vi "SPI API Main.vi"() -> ()   [LabVIEW 2014]
doc: "This example is based on the MAX5216. It allows you to control the voltage output on the SPI chip. This VI interfaces with the SPI Engine on the FPGA."
uses:
  Source/Shared/MCP23S17/Chip Address.ctl
  Source/Shared/MCP23S17/Pin.ctl
  Source/Shared/MCP23S17/Pin Mode.ctl
  Source/Shared/MCP23S17/IOCON BANK 0 Reg Addresses.ctl
  <vilib>/FPGAPlugInAG/cRIO-9081/niLvFpga_Open_cRIO-9081.vi
  <vilib>/rvi/interface/common/dynamic/niFpgaDynamicAddResources.vi
  <vilib>/FPGAPlugInAG/Dynamic/niLvFpga_Reset_Dynamic.vi
  <vilib>/FPGAPlugInAG/Dynamic/niLvFpga_Run_Dynamic.vi
  <vilib>/Utility/error.llb/Error Cluster From Error Code.vi
  <vilib>/rvi/errors/niLvFpgaAdjustHostInterfaceError.vi
  Source/Shared/MCP23S17/Update Mode All Pins.vi
  Source/Shared/MCP23S17/Write Digital All Pins.vi
  Source/Shared/MCP23S17/Write Digital Pin.vi
  Source/Shared/MCP23S17/Update Mode Pin.vi
  Source/Shared/MCP23S17/Update Output Latch All Pins.vi
  Source/Shared/MCP23S17/Update Input Polarity All Pins.vi
  <vilib>/FPGAPlugInAG/Dynamic/niLvFpga_Close_Dynamic.vi
  <vilib>/rvi/interface/nirviOpenFPGA/nirviOpenFPGA.xnode
  FPGA Bitfiles/SPIAPITest_FPGATarget_SPIAPIFPGA_fdd6JLrBLcE.lvbitx
  <vilib>/rvi/interface/nirviMethod/nirviMethod.xnode
  <vilib>/rvi/interface/nirviReadWriteControl/nirviReadWriteControl.xnode
  <vilib>/rvi/interface/nirviCloseFPGA/nirviCloseFPGA.xnode
  <vilib>/rvi/interface/Simulation/niFpgaSimulationCallBeginRW.vi
  NiFpgaLv.dll
  Source/Shared/SLSC configuration Shared.lvlib
  <vilib>/FPGAPlugInAG/Dynamic/niLvFpga_WriteFifo_Dynamic.vi
  <vilib>/rvi/errors/niLvFpgaMergeErrorWithErrorCode.vi
panel:
  in  "Input Polarity":u16 format="%.0b"
  out "Input Polarity Cache":u16 format="%016b"
  out "Output Latch Cache":u16 format="%016b"
  in  "Output Latch":u16 format="%.0b"
  in  "IOCON.BANK = 0 Reg Addresses":T1
  in  "Pin Mode":T2
  out "NC":u64 format="%.0b"
  in  "Pin Value":u8 format="%.0b"
  in  "Pin":T3=1 min=1 max=16
  out "Mode Cache":u16 format="%016b"
  out "Output Cache":u16 format="%016b"
  in  "Value":u16 format="%016b"
  out "SPI Command":u32 format="%.0b"
  out "Transfer Length (bits)":u8
  in  "Mode":u16 format="%016b"
  in  "Chip Address (A2 A1 A0)":T4 max=7
  in  "Message  Type":T5(ring)
  out "Chip Select out":u8
  out "Data to DAC":u64 format="%032b"
  in  "Write":bool
  in  "Chip Select":u8
  out "Binary to DAC":u64
  in  "data rate (S/s)":u32=4000000
  in  "SPI PHY Settings":T6={"Divide Value"=255, "Transfer Length (bits)"=32, "CS Asserted Polarity"=FALSE, "Clock Polarity (CPOL)"=FALSE, "Clock Phase (CPHA)"=FALSE, "Lengthen MISO Setup"=FALSE, "Direction Change Bit"=0, "MOSI Starts as Output"=FALSE, "Tristatable MOSI"=FALSE}
  in  "stop":bool
  # "Overview: This example is based on the MAX5216.  It allows you to control the\nvoltage output on the SPI chip. \nRequirements: LabVIEW Full Development System, LabVIEW Real Time, \nLabVIEW FPGA, MAX5216, NI System on Module, NI 9651.\nInstructions:\n1. The SPI PHY Settings are already setup for the MAX5216.  Do not adjust them.\n2. Plug the MAX5216 into PMOD1 on the NI 9651.\n3. Setup Vref according to the user manual.\n4. Run the VI.\n5. Adjust the Voltage Output and observe the voltage change on the MAX5216."
  # "SPI Settings"
  # "MSB"
  # "LSB"
  # "Sampling Info"
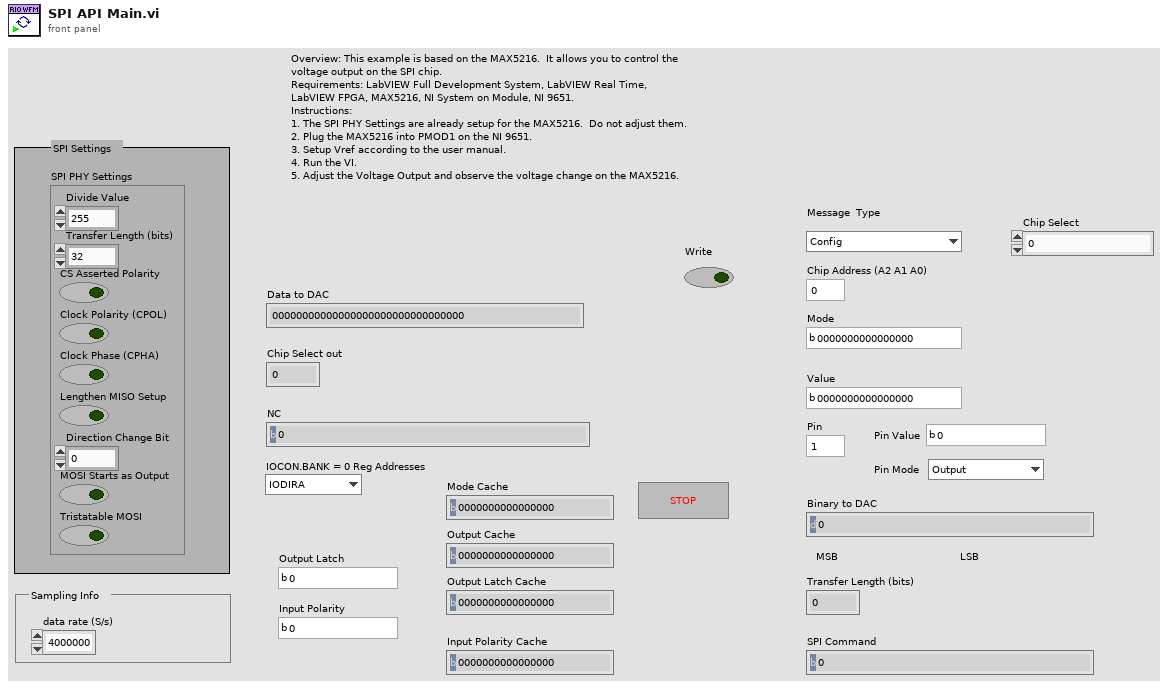
[diagram p1: front panel]
types:
  T1 = typedef "SLSC configuration Shared.lvlib/IOCON BANK 0 Reg Addresses.ctl" = enum8{"IODIRA", "IODIRB", "IPOLA", "IPOLB", "GPINTENA", "GPINTENB", "DEFVALA", "DEFVALB", "INTCONA", "INTCONB", "IOCONA", "IOCONB", "GPPUA", "GPPUB", "INTFA", "INTFB", "INTCAPA", "INTCAPB", "GPIOA", "GPIOB", "OLATA", "OLATB"}
  T2 = typedef "SLSC configuration Shared.lvlib/Pin Mode.ctl" = enum8{"Output", "Input"}
  T3 = typedef "SLSC configuration Shared.lvlib/Pin.ctl" = u8
  T4 = typedef "SLSC configuration Shared.lvlib/Chip Address.ctl" = u8
  T5 = enum16{"Config", "Update Mode All Pins", "Update Mode Pin", "Write Digital All Pins", "Write Digital Pin", "Read Digital Pins", "Read Byte", "Update Output Latches All Pins", "Update Input Polarity All Pins", "Arindam 1", "Arindam 2", "Ardinam 3"}
  T6 = cluster{"Divide Value":u8, "Transfer Length (bits)":u8, "CS Asserted Polarity":bool, "Clock Polarity (CPOL)":bool, "Clock Phase (CPHA)":bool, "Lengthen MISO Setup":bool, "Direction Change Bit":u8, "MOSI Starts as Output":bool, "Tristatable MOSI":bool}
  T7 = typedef "SLSC configuration Shared.lvlib/SPI Command.ctl" = cluster{"SPI Command":u32, "Transfer Length":u8}
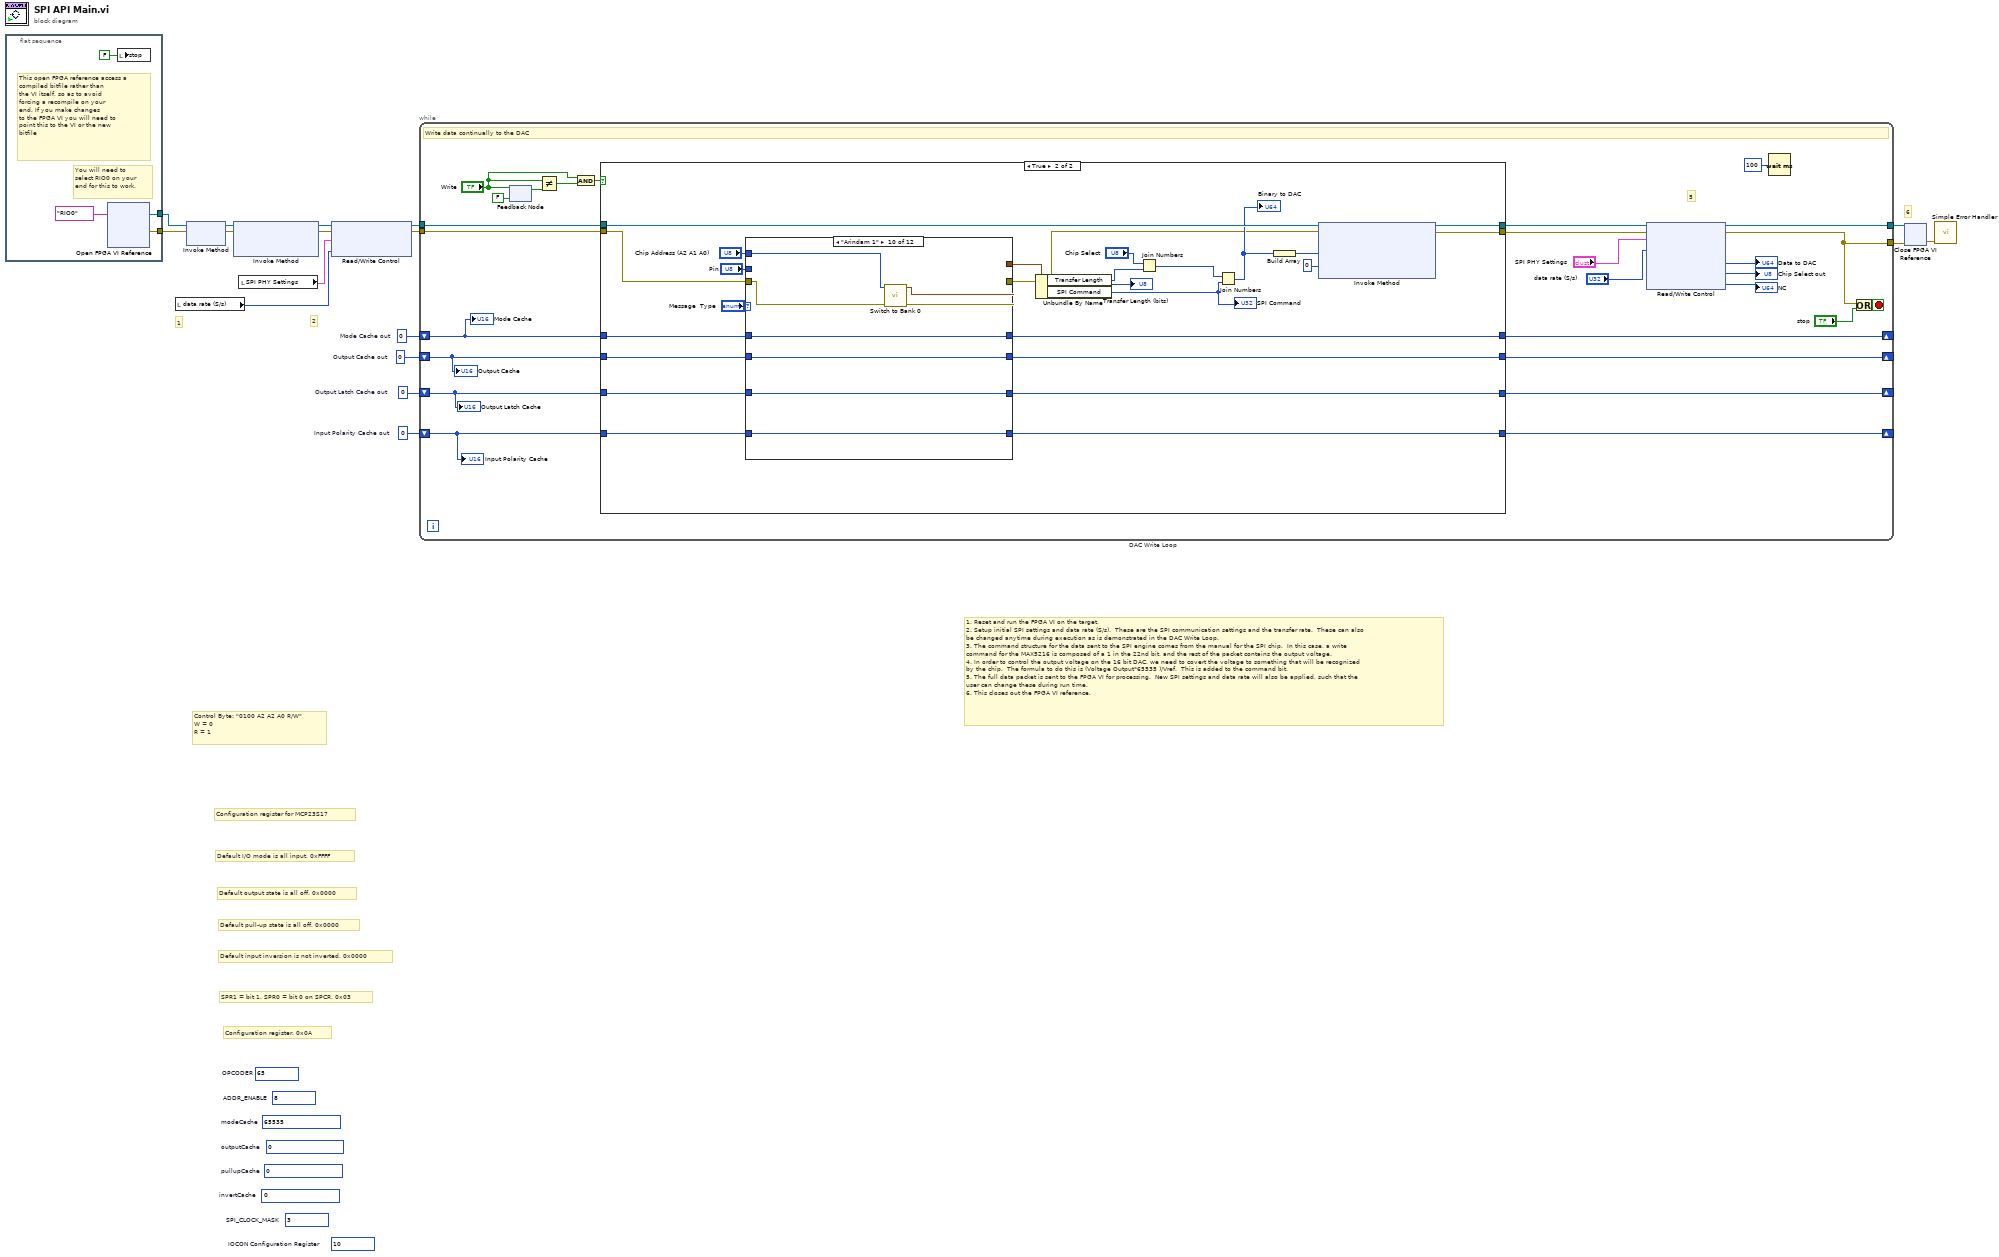
[diagram p0: block diagram]
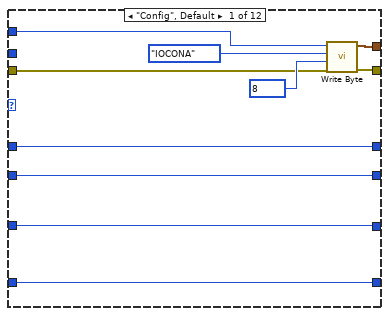
[diagram p3: hidden frame]
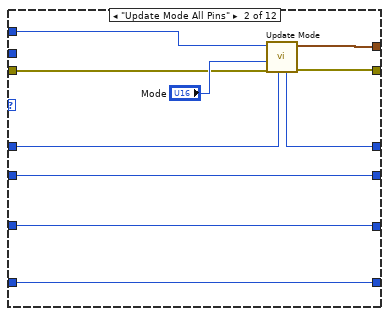
[diagram p4: hidden frame]
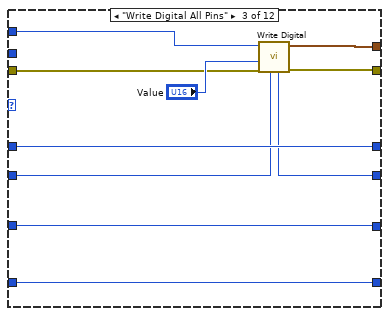
[diagram p5: hidden frame]
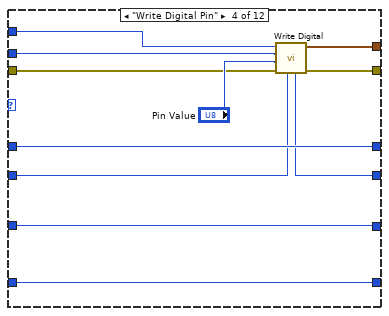
[diagram p6: hidden frame]
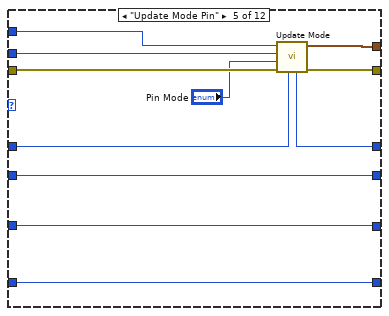
[diagram p7: hidden frame]
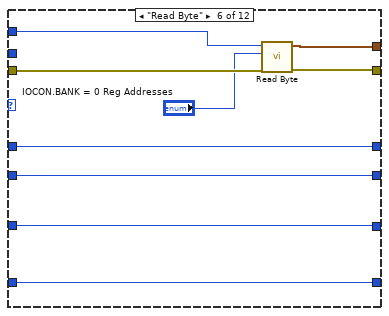
[diagram p8: hidden frame]
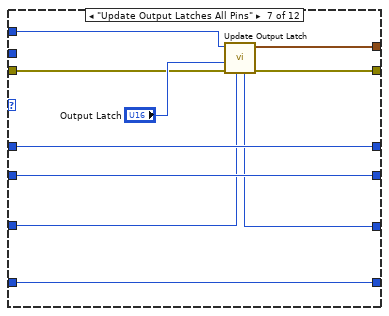
[diagram p9: hidden frame]
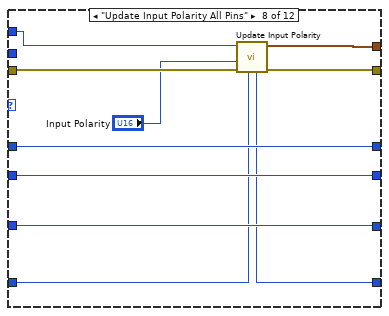
[diagram p10: hidden frame]
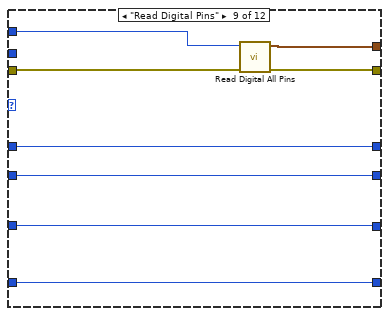
[diagram p11: hidden frame]
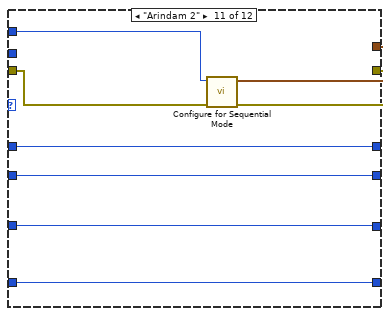
[diagram p12: hidden frame]
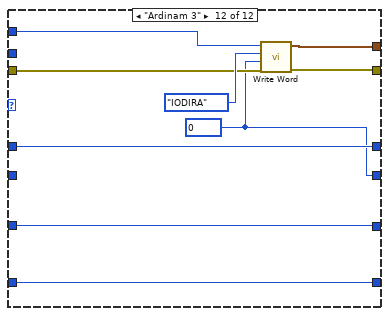
[diagram p13: hidden frame]
diagram:
  w1 = u16 0  # Input Polarity Cache out
  w2 = u16 0  # Output Latch Cache out
  w3 = u16 0  # Output Cache out
  w4 = u16 0  # Mode Cache out
  (unwired) u8 10  # IOCON Configuration Register
  (unwired) u8 3  # SPI_CLOCK_MASK
  (unwired) u16 0  # invertCache
  (unwired) u16 0  # pullupCache
  (unwired) u16 0  # outputCache
  (unwired) u16 65535  # modeCache
  (unwired) u8 8  # ADDR_ENABLE
  (unwired) u8 65  # OPCODER
  # "Configuration register, 0x0A"
  # "SPR1 = bit 1, SPR0 = bit 0 on SPCR, 0x03"
  # "Default input inversion is not inverted, 0x0000"
  # "Default pull-up state is all off, 0x0000"
  # "Default output state is all off, 0x0000"
  # "Default I/O mode is all input, 0xFFFF"
  # "Configuration register for MCP23S17"
  # "Control Byte: \"0100 A2 A2 A0 R/W\"\nW = 0\nR = 1"
  # "1. Reset and run the FPGA VI on the target.\n2. Setup initial SPI settings and data rate (S/s).  These are the SPI communication settings and the transfer rate.  These can also\nbe changed anytime during execution as is demonstrated in the DAC Write Loop.\n3. The command structure for the data sent to the SPI engine comes from the manual for the SPI chip.  In this case, a write\ncommand for the MAX5216 is composed of a 1 in the 22nd bit, and the rest of the packet contains the output voltage.\n4. In order to control the output voltage on the 16 bit DAC, we need to covert the voltage to something that will be recognized\nby the chip.  The formula to do this is (Voltage Output*65535 )/Vref.  This is added to the command bit.\n5. The full data packet is sent to the FPGA VI for processing.  New SPI settings and data rate will also be applied, such that the\nuser can change these during run time.\n6. This closes out the FPGA VI reference."
  # "6"
  # "2"
  # "1"
  n1 = flat-sequence {
    tunnel: [w20] -> w17
    tunnel: [w19] -> w16
    frame #0 {
      # "You will need to\nselect RIO0 on your\nend for this to work."
      # "This open FPGA reference access a\ncompiled bitfile rather than \nthe VI itself, so as to avoid\nforcing a recompile on your\nend. If you make changes\nto the FPGA VI you will need to\npoint this to the VI or the new\nbitfile"
      n2 = xnode "Open FPGA VI Reference"("resource name"=tag "RIO0") -> ("FPGA VI Reference Out"=w20:refnum<k20>, "error out"=w19:errorcluster)  [unwired: 1 in]
      n3 = local write "stop"(FALSE ("stop")) -> ()
    }
  }
  n4 = local read "data rate (S/s)"() -> (w5:u32)
  n5 = xnode "Invoke Method"("FPGA VI Reference In"=w17, "error in"=w16) -> ("FPGA VI Reference Out"=w11:refnum<k20>, "error out"=w10:errorcluster)
  n6 = xnode "Invoke Method"("FPGA VI Reference In"=w11, "error in"=w10) -> ("FPGA VI Reference Out"=w12:refnum<k20>, "error out"=w14:errorcluster)  [unwired: 1 in]
  n7 = local read "SPI PHY Settings"() -> (w8:T6)
  n8 = xnode "Read/Write Control"("FPGA VI Reference In"=w12, "error in"=w14, "SPI PHY Settings"=w8, "Sample Rate (S/s)"=w5) -> ("FPGA VI Reference Out"=w9:refnum<k20>, "error out"=w13:errorcluster)
  n9 = while "DAC Write Loop" {
    tunnel: w9 -> [w46]
    tunnel: w13 -> [w47]
    tunnel: [w40] -> w7
    tunnel: [w39] -> w6
    shift-right: [w29] -> _
    shift-left: w4 -> [w30]
    shift-right: [w27] -> _
    shift-left: w3 -> [w28]
    shift-right: [w24] -> _
    shift-left: w2 -> [w25]
    shift-right: [w22] -> _
    shift-left: w1 -> [w23]
    stop <- w48 stop-if-true
    # "5"
    # "Write data continually to the DAC"
    n10 = feedback-in #1("Write") -> ()
    n11 = feedback #1(FALSE ("Write")) -> (w36:bool)
    n12 = Not Equal?(x="Write", y=w36) -> (x != y?=w33:bool)
    n13 = And(x="Write", y=w33) -> (x .and. y?=w34:bool)
    n14 = case shown="True" w34 {
      tunnel: w47 -> [w54 w63]
      tunnel: w46 -> [w53 w78]
      tunnel: [w53 w77] -> w42
      tunnel: [w54 w76] -> w41
      tunnel: w30 -> [w52 w69]
      tunnel: [w52 w68] -> w29
      tunnel: w28 -> [w51 w67]
      tunnel: [w51 w66] -> w27
      tunnel: w25 -> [w50 w61]
      tunnel: [w50 w60] -> w24
      tunnel: w23 -> [w49 w59]
      tunnel: [w49 w58] -> w22
      frame False {
      }
      frame True {
        n15 = case shown="\"Arindam 1\"" "Message  Type" {
          tunnel: [w88 w98 w108 w117 w129 w134 w148 w157 w166 w168 w176 w191] -> w57
          tunnel: w69 -> [w84 w92 w105 w119 w124 w136 w144 w153 w165 w174 w182 w189]
          tunnel: [w84 w91 w105 w119 w123 w136 w144 w153 w165 w174 w182 w189] -> w68
          tunnel: w67 -> [w83 w95 w103 w113 w128 w135 w143 w152 w164 w173 w181 _]
          tunnel: [w83 w95 w102 w114 w128 w135 w143 w152 w164 w173 w181 w184] -> w66
          tunnel: "Chip Address (A2 A1 A0)" -> [w87 w97 w107 w118 w130 w139 w149 w158 w167 w175 w183 w192]
          tunnel: "Pin" -> [_ _ _ w116 w127 _ _ _ _ _ _ _]
          tunnel: w63 -> [w82 w93 w104 w112 w126 w138 w146 w155 w163 w172 w180 w188]
          tunnel: [w81 w94 w101 w111 w125 w137 w145 w156 w162 w171 w179 w187] -> w62
          tunnel: w61 -> [w80 w90 w100 w110 w121 w132 w142 w159 w161 w170 w178 w186]
          tunnel: [w80 w90 w100 w110 w121 w132 w141 w159 w161 w170 w178 w186] -> w60
          tunnel: w59 -> [w79 w89 w99 w109 w120 w131 w140 w151 w160 w169 w177 w185]
          tunnel: [w79 w89 w99 w109 w120 w131 w140 w150 w160 w169 w177 w185] -> w58
          frame "Config", Default {
            n16 = call "Write Byte.vi"("error in (no error)"=w82, "Value"=u8 8, "Reg Address"=IOCON_BANK_0_Reg_Addresses."IOCONA", "Chip Address (A2 A1 A0)"=w87) -> ("error out"=w81:errorcluster, "SPI Command"=w88:T7)  [unwired: 6 in]
          }
          frame "Update Mode All Pins" {
            n17 = call-poly "Update Mode.vi"("Mode Cache in"=w92, "error in (no error)"=w93, "Mode"="Mode", "Chip Address (A2 A1 A0)"=w97) -> ("error out"=w94:errorcluster, "SPI Command"=w98:T7, "Mode Cache out"=w91:u16)  [unwired: 5 in]
          }
          frame "Write Digital All Pins" {
            n18 = call-poly "Write Digital.vi"("Output Cache in"=w103, "error in (no error)"=w104, "Value"="Value", "Chip Address (A2 A1 A0)"=w107) -> ("error out"=w101:errorcluster, "SPI Command"=w108:T7, "Output Cache out"=w102:u16)  [unwired: 5 in]
          }
          frame "Write Digital Pin" {
            n19 = call-poly "Write Digital.vi"("Output Cache in"=w113, "error in (no error)"=w112, "Value"="Pin Value", "Pin"=w116, "Chip Address (A2 A1 A0)"=w118) -> ("error out"=w111:errorcluster, "SPI Command"=w117:T7, "Output Cache out"=w114:u16)  [unwired: 4 in]
          }
          frame "Update Mode Pin" {
            n20 = call-poly "Update Mode.vi"("Mode Cache in"=w124, "error in (no error)"=w126, "Mode"="Pin Mode", "Pin"=w127, "Chip Address (A2 A1 A0)"=w130) -> ("error out"=w125:errorcluster, "SPI Command"=w129:T7, "Mode Cache out"=w123:u16)  [unwired: 4 in]
          }
          frame "Read Byte" {
            n21 = call "Read Byte.vi"("error in (no error)"=w138, "IOCON.BANK = 0 Reg Addresses"="IOCON.BANK = 0 Reg Addresses", "Chip Address (A2 A1 A0)"=w139) -> ("error out"=w137:errorcluster, "SPI Command"=w134:T7)  [unwired: 7 in]
          }
          frame "Update Output Latches All Pins" {
            n22 = call-poly "Update Output Latch.vi"("Output Latch Cache in"=w142, "error in (no error)"=w146, "Output Latch"="Output Latch", "Chip Address (A2 A1 A0)"=w149) -> ("error out"=w145:errorcluster, "SPI Command"=w148:T7, "Output Latch Cache out"=w141:u16)  [unwired: 5 in]
          }
          frame "Update Input Polarity All Pins" {
            n23 = call-poly "Update Input Polarity.vi"("Input Polarity Cache in"=w151, "error in (no error)"=w155, "Input Polarity"="Input Polarity", "Chip Address (A2 A1 A0)"=w158) -> ("error out"=w156:errorcluster, "SPI Command"=w157:T7, "Input Polarity Cache out"=w150:u16)  [unwired: 5 in]
          }
          frame "Read Digital Pins" {
            n24 = call "Read Digital All Pins.vi"("error in (no error)"=w163, "Chip Address (A2 A1 A0)"=w167) -> ("error out"=w162:errorcluster, "SPI Command"=w166:T7)  [unwired: 8 in]
          }
          frame "Arindam 1" {
            n25 = call "Switch to Bank 0.vi"("error in (no error)"=w172, "Chip Address (A2 A1 A0)"=w175) -> ("error out"=w171:errorcluster, "SPI Command"=w168:T7)  [unwired: 8 in]
          }
          frame "Arindam 2" {
            n26 = call "Configure for Sequential Mode.vi"("error in (no error)"=w180, "Chip Address (A2 A1 A0)"=w183) -> ("error out"=w179:errorcluster, "SPI Command"=w176:T7)  [unwired: 8 in]
          }
          frame "Ardinam 3" {
            w184 = u16 0 ("Value")
            n27 = call "Write Word.vi"("error in (no error)"=w188, "Value"=w184, "Reg Address"=IOCON_BANK_0_Reg_Addresses."IODIRA", "Chip Address (A2 A1 A0)"=w192) -> ("error out"=w187:errorcluster, "SPI Command"=w191:T7)  [unwired: 6 in]
          }
        }
        n28 = Unbundle By Name(w57) -> ("Transfer Length"=w56:u8, "SPI Command"=w55:u32)
        "Transfer Length (bits)" <- w56
        "SPI Command" <- w55
        n29 = Join Numbers(hi="Chip Select", lo=w56) -> ((hi.lo)=w71:u16)
        n30 = Join Numbers(hi=w71, lo=w55) -> ((hi.lo)=w74:u64)
        "Binary to DAC" <- w74
        n31 = Build Array(w74) -> (w75:u64[])
        n32 = xnode "Invoke Method"("FPGA VI Reference In"=w78, "error in"=w62, "Data"=w75, "Timeout (ms)"=0) -> ("FPGA VI Reference Out"=w77:refnum<k20>, "error out"=w76:errorcluster)  [unwired: 1 out]
      }
    }
    n33 = xnode "Read/Write Control"("FPGA VI Reference In"=w42, "error in"=w41, "SPI PHY Settings"="SPI PHY Settings", "Sample Rate (S/s)"="data rate (S/s)") -> ("FPGA VI Reference Out"=w40:refnum<k20>, "error out"=w39:errorcluster, "Data to DAC"=→"Data to DAC":u64, "Chip Select"=→"Chip Select out":u8, "NC"=→"NC":u64)
    n34 = Wait (ms)(milliseconds to wait=u32 100) -> ()  [unwired: 1 out]
    n35 = Or(x=w39, y="stop") -> (x .or. y?=w48:bool)
    "Output Cache" <- w28
    "Mode Cache" <- w30
    "Output Latch Cache" <- w25
    "Input Polarity Cache" <- w23
  }
  n36 = xnode "Close FPGA VI Reference"("FPGA VI Reference In"=w7, "error in"=w6) -> ("error out"=w15:errorcluster)
  n37 = call <vilib>:"Simple Error Handler.vi"("error in (no error)"=w15) -> ()  [unwired: 1 in, 8 out]
